vi "SVN_Log_ParseCMDOutput.vi"(8 "Error In":errorcluster, 11 "SVN_Log_XML (In)":string="<?xml version=\"1.0\" encoding=\"UTF-8\"?>\r\n<log>\r\n<logentry\r\n   revision=\"23\">\r\n<author>Admin</author>\r\n<date>2018-04-07T20:16:29.107705Z</date>\r\n<msg></msg>\r\n</logentry>\r\n<logentry\r\n   revision=\"22\">\r\n<author>Admin</author>\r\n<date>2018-04-07T20:12:54.923454Z</date>\r\n<msg></msg>\r\n</logentry>\r\n<logentry\r\n   revision=\"21\">\r\n<author>Admin</author>\r\n<date>2018-04-07T20:12:03.070489Z</date>\r\n<msg></msg>\r\n</logentry>\r\n<logentry\r\n   revision=\"20\">\r\n<author>Marvin</author>\r\n<date>2017-12-05T21:00:12.256074Z</date>\r\n<msg></msg>\r\n</logentry>\r\n<logentry\r\n   revision=\"17\">\r\n<author>Marvin</author>\r\n<date>2017-12-05T20:36:10.326601Z</date>\r\n<msg>10k LoadSpeedTest\r\n</msg>\r\n</logentry>\r\n<logentry\r\n   revision=\"16\">\r\n<author>Marvin</author>\r\n<date>2017-07-06T14:47:03.129259Z</date>\r\n<msg></msg>\r\n</logentry>\r\n<logentry\r\n   revision=\"11\">\r\n<author>Marvin</author>\r\n<date>2017-07-04T16:12:46.837966Z</date>\r\n<msg></msg>\r\n</logentry>\r\n<logentry\r\n   revision=\"7\">\r\n<author>Marvin</author>\r\n<date>2017-07-04T16:05:39.382517Z</date>\r\n<msg></msg>\r\n</logentry>\r\n<logentry\r\n   revision=\"6\">\r\n<author>Marvin</author>\r\n<date>2017-07-04T16:05:05.356571Z</date>\r\n<msg></msg>\r\n</logentry>\r\n<logentry\r\n   revision=\"3\">\r\n<author>Marvin</author>\r\n<date>2017-07-04T15:57:28.132419Z</date>\r\n<msg></msg>\r\n</logentry>\r\n<logentry\r\n   revision=\"1\">\r\n<author>Marvin</author>\r\n<date>2017-07-04T15:51:57.071483Z</date>\r\n<msg>Imported folder structure</msg>\r\n</logentry>\r\n</log>\r\n") -> (0 "Error Out":errorcluster, 3 "SVN Log-Info_Cluster[]":T1[](array[typedef]))   [LabVIEW 2014]
uses:
  <resource>/objmgr/DOMUserDefRef.rc
  <vilib>/xml/NI_XML.lvlib
  controls/SVN_LogEntry_Cluster.ctl
  <vilib>/xml/Load XML String.vi
panel:
  out "Array 5":string[](array[string])
  out "Array 4":i32[](array[ring]) items=["Element_Node"=1, "Attribute_Node"=2, "Text_Node"=3, "CDATASection_Node"=4, "EntityReference_Node"=5, "Entity_Node"=6, "ProcessingInstruction_Node"=7, "Comment_Node"=8, "Document_Node"=9, "DocumentType_Node"=10, "DocumentFragment_Node"=11, "Notation_Node"=12]
  out "Array 3":string[](array[string])
  out "Array 2":string[](array[string])
  out "Array":errorcluster[](array[cluster])
  out "Node Type":i32(ring)=1 items=["Element_Node"=1, "Attribute_Node"=2, "Text_Node"=3, "CDATASection_Node"=4, "EntityReference_Node"=5, "Entity_Node"=6, "ProcessingInstruction_Node"=7, "Comment_Node"=8, "Document_Node"=9, "DocumentType_Node"=10, "DocumentFragment_Node"=11, "Notation_Node"=12]
  out "node text":string
  out "Node Value":string
  out "Node Name":string
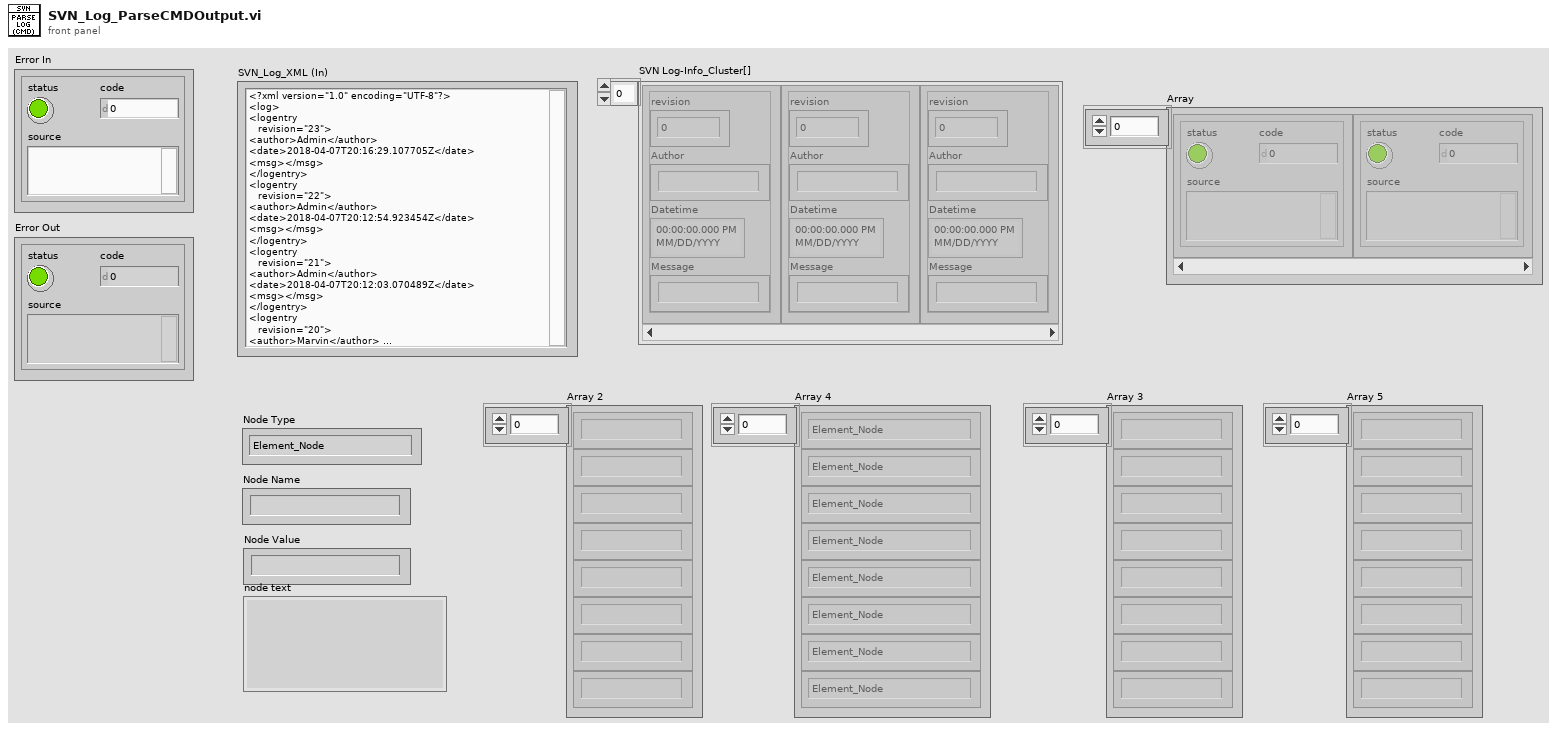
[diagram p1: front panel]
types:
  T1 = typedef "SVN_LogEntry_Cluster.ctl" = cluster{"revision":i32, "Author":string, "Datetime":timestamp, "Message":string}
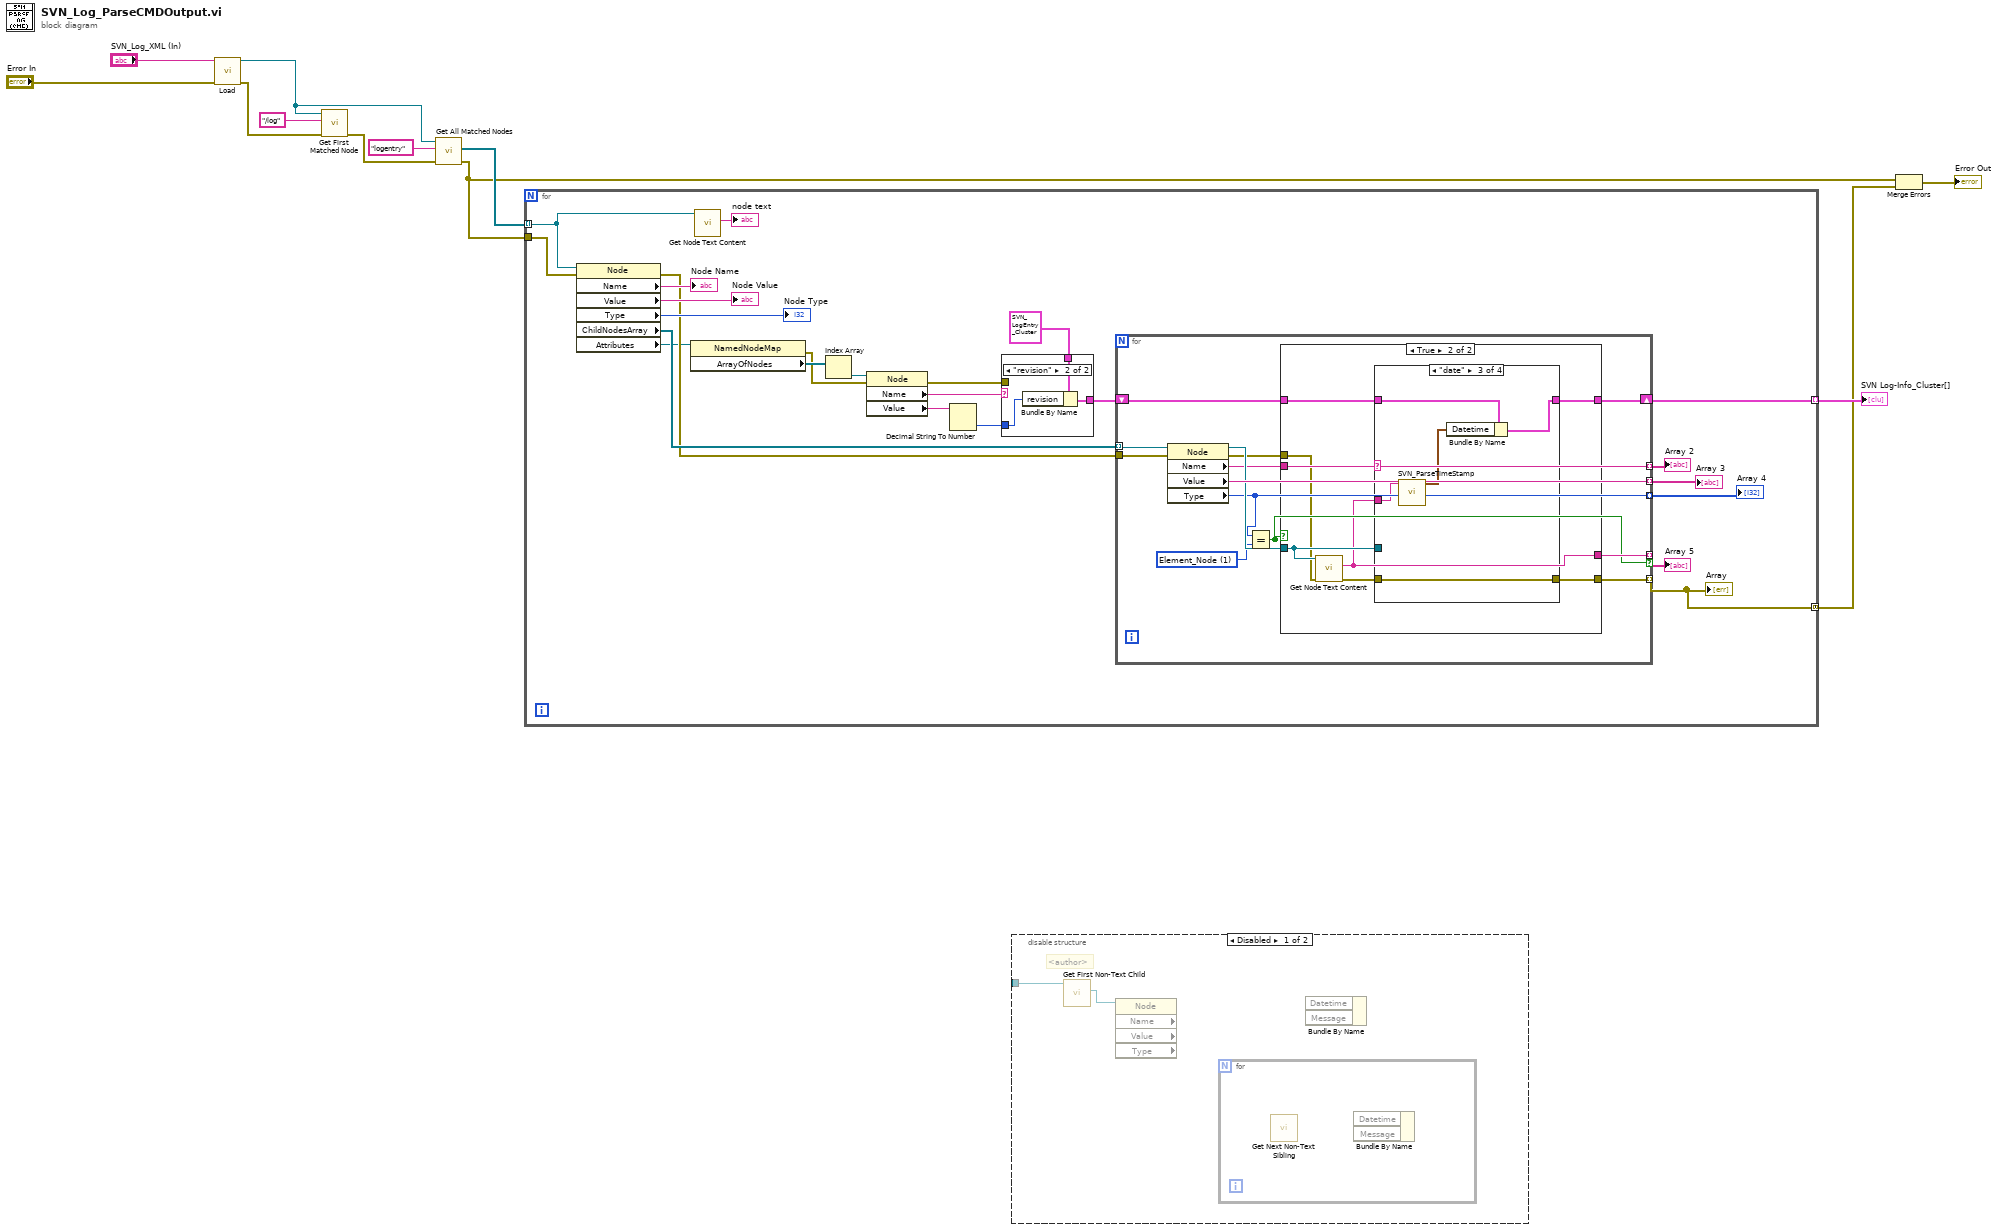
[diagram p0: block diagram]
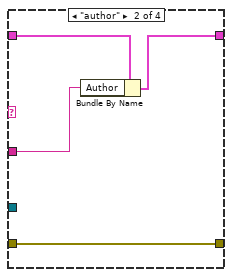
[diagram p5: hidden frame]
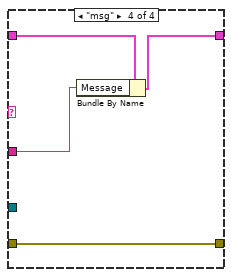
[diagram p6: hidden frame]
diagram:
  n1 = call-poly <vilib>:"Load.vi"("XML string"="SVN_Log_XML (In)", "error in (no error)"="Error In") -> ("DOM document out"=w10:refnum<k20>, "error out"=w5:errorcluster)  [unwired: 11 in, 1 out]
  n2 = call <vilib>:"Get First Matched Node.vi"("error in (no error)"=w5, "XPath expression"="/log", "node in"=w10) -> ("error out"=w4:errorcluster)  [unwired: 6 in, 2 out]
  n3 = call <vilib>:"Get All Matched Nodes.vi"("error in (no error)"=w4, "XPath expression"="logentry", "node in"=w10) -> ("error out"=w1:errorcluster, "node result array"=w9:refnum<k20>[])  [unwired: 6 in, 1 out]
  n4 = for {
    tunnel: w9 -> [w22] mode=indexing
    tunnel: [w27] -> w8 mode=indexing
    tunnel: w1 -> [w26]
    tunnel: [w24] -> w3 mode=concatenating
    n5 = property class="Node"(reference=w22, error in=w26) -> (error out=w25:errorcluster, "Name"=→"Node Name":string, "Value"=→"Node Value":string, "Type"=→"Node Type":i32, "ChildNodesArray"=w32:refnum<k20>[], "Attributes"=w23:refnum<k20>)  [unwired: 1 out]
    n6 = property class="NamedNodeMap"(reference=w23) -> (error out=w14:errorcluster, "ArrayOfNodes"=w21:refnum<k20>[])  [unwired: 1 in, 1 out]
    n7 = call <vilib>:"Get Node Text Content.vi"("node in"=w22) -> ("node text"=→"node text":string)  [unwired: 8 in, 2 out]
    n8 = Index Array(array=w21) -> (element=w20:refnum<k20>)  [unwired: 1 in]
    n9 = property class="Node"(reference=w20, error in=w14) -> (error out=w13:errorcluster, "Name"=w15:string, "Value"=w17:string)  [unwired: 1 out]
    n10 = Decimal String To Number(string=w17) -> (number=w16:i32)  [unwired: 2 in, 1 out]
    n11 = case shown="\"revision\"" w15 {
      tunnel: T1 {"revision"=0, "Author"="", "Datetime"=timestamp(0 s since 1904-01-01), "Message"=""} -> [w37 w40]
      tunnel: [w37 w39] -> w18
      tunnel: w16 -> [_ w38]
      tunnel: w13 -> [_ _]
      frame "", Default {
      }
      frame "revision" {
        n12 = Bundle By Name(cluster=w40, "revision"=w38) -> (w39:T1)
      }
    }
    n13 = for {
      tunnel: w32 -> [w53] mode=indexing
      tunnel: [w41] -> w24 mode=indexing
      tunnel: [w45] -> w31 mode=indexing
      tunnel: [w52] -> w30 mode=indexing
      tunnel: [w49] -> w29 mode=indexing
      tunnel: [w50] -> w28 mode=indexing if=w47
      shift-right: [w44] -> w27
      shift-left: w18 -> [w46]
      tunnel: w25 -> [w43]
      w48 = 1 items=["Element_Node"=1, "Attribute_Node"=2, "Text_Node"=3, "CDATASection_Node"=4, "EntityReference_Node"=5, "Entity_Node"=6, "ProcessingInstruction_Node"=7, "Comment_Node"=8, "Document_Node"=9, "DocumentType_Node"=10, "DocumentFragment_Node"=11, "Notation_Node"=12] ("Node Type")
      n14 = property class="Node"(reference=w53, error in=w43) -> (reference out=w51:refnum<k20>, error out=w42:errorcluster, "Name"=w45:string, "Value"=w52:string, "Type"=w49:i32)
      n15 = Equal?(x=w49, y=w48) -> (x = y?=w47:bool)
      n16 = case shown="True" w47 {
        tunnel: w51 -> [_ w63]
        tunnel: [_ w59] -> w50
        tunnel: w46 -> [w55 w62]
        tunnel: w45 -> [_ w61]
        tunnel: [w55 w60] -> w44
        tunnel: w42 -> [w54 w58]
        tunnel: [w54 w57] -> w41
        frame False {
        }
        frame True {
          n17 = call <vilib>:"Get Node Text Content.vi"("error in (no error)"=w58, "node in"=w63) -> ("error out"=w56:errorcluster, "node text"=w59:string)  [unwired: 7 in, 1 out]
          n18 = case shown="\"date\"" w61 {
            tunnel: w63 -> [_ _ _ _]
            tunnel: w62 -> [w65 w69 w74 w78]
            tunnel: [w65 w68 w73 w77] -> w60
            tunnel: w59 -> [_ w67 w72 w76]
            tunnel: [w64 w66 w70 w75] -> w57
            tunnel: w56 -> [w64 w66 w70 w75]
            frame "", Default {
            }
            frame "author" {
              n19 = Bundle By Name(cluster=w69, "Author"=w67) -> (w68:T1)
            }
            frame "date" {
              n20 = call "SVN_ParseTimeStamp.vi"("Timestring (In)"=w72) -> ("Timestamp (Out)"=w71:timestamp)  [unwired: 10 in]
              n21 = Bundle By Name(cluster=w74, "Datetime"=w71) -> (w73:T1)
            }
            frame "msg" {
              n22 = Bundle By Name(cluster=w78, "Message"=w76) -> (w77:T1)
            }
          }
        }
      }
    }
    "Array" <- w24
    "Array 2" <- w31
    "Array 3" <- w30
    "Array 4" <- w29
    "Array 5" <- w28
  }
  "SVN Log-Info_Cluster[]" <- w8
  n23 = disable-structure shown="Disabled" {
    disable-tunnel: _ -> [w80 _]
    frame Disabled {
      # "<author>"
      n24 = call <vilib>:"Get First Non-Text Child.vi"("node in"=w80) -> ("child node"=w79:refnum<k20>)  [unwired: 7 in, 3 out]
      n25 = property class="Node" props=["Name", "Value", "Type"](reference=w79) -> ()  [unwired: 1 in, 5 out]
      n26 = for {
        n27 = call <vilib>:"Get Next Non-Text Sibling.vi"() -> ()  [unwired: 8 in, 4 out]
        n28 = Bundle By Name() -> ()  [unwired: 3 in, 1 out]
      }
      n29 = Bundle By Name() -> ()  [unwired: 3 in, 1 out]
    }
    frame Enabled {
    }
  }
  n30 = Merge Errors(w1, w3) -> (→"Error Out":errorcluster)
